vi "Do This.vi"(8 "error in (no error)":errorcluster, 10 "Status Events":refnum<class "Status Events.lvclass">, 11 "VI Analyzer in":refnum<class "VI Analyzer.lvclass">) -> (0 "error out":errorcluster, 3 "VI Analyzer out":refnum<class "VI Analyzer.lvclass">)   [LabVIEW 2014, in "VI Analyzer.lvclass"]
uses:
  VI Analyzer.lvclass
  Classes/Status Events/Status Events.lvclass
  Classes/Job/Job.lvclass/Job.ctl
  VI Analyzer.lvclass/VI Analyzer.ctl
  <vilib>/Utility/error.llb/DialogType.ctl
  <vilib>/addons/analyzer/NI_VIAnalyzerTKVIs.lvlib
  Classes/Job/Job.lvclass
  JUnit/VI Analyzer Parsing.lvlib
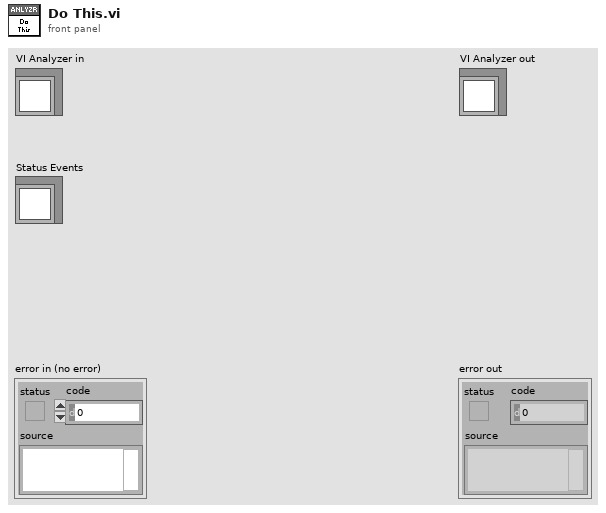
[diagram p1: front panel]
types:
  T1 = typedef "VIAnAPI Ref.ctl" = refnum<k1>
  T2 = typedef "VIAnCtl Results.ctl" = cluster{"Test Name":string, "Results Data":T3[], "Status":T4, "Exceed Max Fails?":bool}
  T3 = typedef "VIAnCtl ResultsData (index).ctl" = cluster{"Result Message":string, "Ref Index":i32}
  T4 = typedef "VIAnCtl ResultStatus.ctl" = enum16{"Pass", "Fail", "Skipped", "VI not loadable", "Test not loadable", "Test not runnable", "Test error out"}
  T5 = typedef "VIAnRes Parsed Results Data (by VI).ctl" = cluster{"VI Path":path, "Pass":cluster{"row":i32, "column":i32}[], "Fail":cluster{"row":i32, "column":i32}[], "Skipped":cluster{"row":i32, "column":i32}[], "VI not loadable":cluster{"row":i32, "column":i32}[], "Test not loadable":cluster{"row":i32, "column":i32}[], "Test not runnable":cluster{"row":i32, "column":i32}[], "Test error out":cluster{"row":i32, "column":i32}[]}
  T6 = typedef "VIAnRes Parsed Results Data (by Test).ctl" = cluster{"Test Name":string, "Pass":cluster{"VI Path":path, "index":cluster{"row":i32, "column":i32}}[], "Fail":cluster{"VI Path":path, "index":cluster{"row":i32, "column":i32}}[], "Skipped":cluster{"VI Path":path, "index":cluster{"row":i32, "column":i32}}[]}
  T7 = typedef "VIAnCtl Test Config Data.ctl" = cluster{"Test Name":string, "Config Ref":refnum<vi>, "Ref Valid?":bool, "Test Ranking":T8, "Max Failures":u32, "Test Path":path, "Control Values":T9[], "Selected?":bool}
  T8 = typedef "VIAnCtl TestRanking.ctl" = u16
  T9 = typedef "VIAnCtl Config Control Value.ctl" = cluster{"Control Name":string, "Control Value":variant}
  T10 = cluster{"Raw Results":T2[][], "Parsed Results Data (by VI)":T5[], "Parsed Results Data (by Test)":T6[], "Summary Statistics":cluster{"Passed Tests":i32, "Failed Tests":i32, "Skipped Tests":i32, "VIs not loadable":i32, "Tests not loadable":i32, "Tests not runnable":i32, "Test error out":i32, "Start Time":u32, "Total Time (s)":dbl}, "Test Config Data":T7[]}
  T11 = cluster{"Passed Tests":i32, "Failed Tests":i32, "Skipped Tests":i32, "VIs not loadable":i32, "Tests not loadable":i32, "Tests not runnable":i32, "Test error out":i32, "Start Time":u32, "Total Time (s)":dbl}
  T12 = typedef "DialogType.ctl" = u16
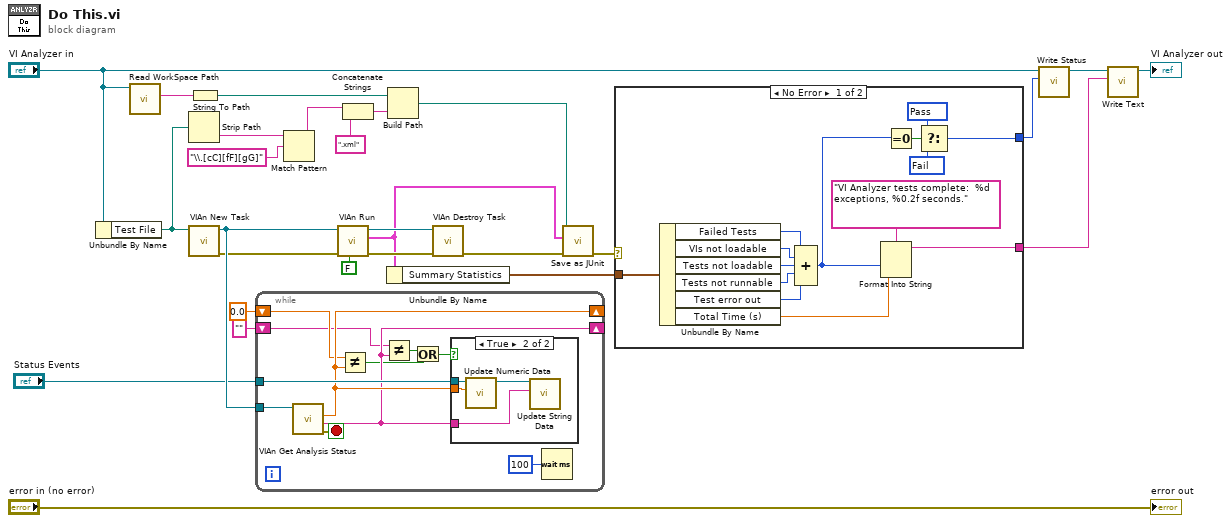
[diagram p0: block diagram]
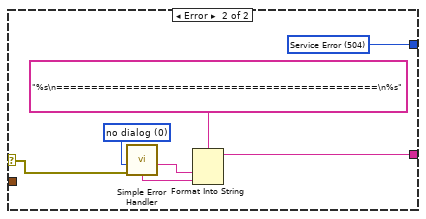
[diagram p2: hidden frame]
diagram:
  n1 = Unbundle By Name("VI Analyzer in") -> ("Test File"=w23:path)
  n2 = call "Read WorkSpace Path.vi"("Job in"="VI Analyzer in") -> ("WorkSpace Path"=w20:string)  [unwired: 8 in, 2 out]
  n3 = Strip Path(path=w23) -> (name=w21:string)  [unwired: 1 out]
  n4 = call <vilib>:"VIAn New Task.vi"("Path to Configuration File"=w23) -> ("error out"=w15:errorcluster, "VI Analyzer Task out"=w26:T1)  [unwired: 2 in, 7 out]
  n5 = String To Path(string=w20) -> (path=w19:path)
  n6 = while {
    tunnel: w26 -> [w36]
    tunnel: "Status Events" -> [w35]
    shift-right: [w34] -> _
    shift-left: 0.0 ("Percent Complete") -> [w33]
    shift-right: [w32] -> _
    shift-left: "" ("VI in Analysis") -> [w31]
    stop <- w37 stop-if-true
    n7 = call <vilib>:"VIAn Get Analysis Status.vi"("VI Analyzer Task in"=w36) -> ("error out"=w37:errorcluster, "VI in Analysis"=w32:string, "Percent Complete"=w34:dbl)  [unwired: 1 in, 7 out]
    n8 = Not Equal?(x=w33, y=w34) -> (x != y?=w29:bool)
    n9 = Not Equal?(x=w31, y=w32) -> (x != y?=w30:bool)
    n10 = Or(x=w30, y=w29) -> (x .or. y?=w28:bool)
    n11 = case shown="True" w28 {
      tunnel: w35 -> [_ w42]
      tunnel: w34 -> [_ w40]
      tunnel: w32 -> [_ w39]
      frame False {
      }
      frame True {
        n12 = call "Update Numeric Data.vi"("Numeric Data"=w40, "Status Updater in"=w42) -> ("Status Updater out"=w41:refnum<class "Status Events.lvclass">)  [unwired: 8 in, 1 out]
        n13 = call "Update String Data.vi"("String Data"=w39, "Status Updater in"=w41) -> ()  [unwired: 8 in, 2 out]
      }
    }
    n14 = Wait (ms)(milliseconds to wait=u32 100) -> ()  [unwired: 1 out]
  }
  n15 = Match Pattern(string=w21, regular expression="\\.[cC][fF][gG]") -> (before substring=w18:string)  [unwired: 1 in, 3 out]
  n16 = call <vilib>:"VIAn Run.vi"("Show Results Window?"=FALSE, "error in (no error)"=w15, "VI Analyzer Task in"=w26) -> ("error out"=w14:errorcluster, "Analysis Results"=w1:T10, "VI Analyzer Task out"=w27:T1)  [unwired: 6 out]
  n17 = Concatenate Strings(w18, ".xml" ("string")) -> (w8:string)
  n18 = Unbundle By Name(w1) -> ("Summary Statistics"=w16:T11)
  n19 = Build Path(base path=w19, name or relative path=w8) -> (appended path=w2:path)
  n20 = call <vilib>:"VIAn Destroy Task.vi"("error in (no error)"=w14, "VI Analyzer Task in"=w27) -> ("error out"=w3:errorcluster)  [unwired: 9 out]
  n21 = call "Save as JUnit.vi"("Error In (No Error)"=w3, "Analysis Results"=w1, "XML file path"=w2) -> ("Error Out"=w4:errorcluster)  [unwired: 8 in]
  n22 = case shown="No Error" w4 {
    selector: w4 -> [_ w58]
    tunnel: w16 -> [w56 _]
    tunnel: [w43 w63] -> w13
    tunnel: [w48 w57] -> w12
    frame No Error {
      w46 = u16 200 items=["Service Error"=504, "Abort"=503, "Fail"=500, "Pass"=200] ("Status")
      w47 = u16 500 items=["Service Error"=504, "Abort"=503, "Fail"=500, "Pass"=200] ("Status")
      n23 = Unbundle By Name(w56) -> ("Failed Tests"=w52:i32, "VIs not loadable"=w51:i32, "Tests not loadable"=w55:i32, "Tests not runnable"=w54:i32, "Test error out"=w53:i32, "Total Time (s)"=w49:dbl)
      n24 = Compound Arithmetic op=ADD(w52, w51, w55, w54, w53) -> (w45:i32)
      n25 = Format Into String(format string="VI Analyzer tests complete:  %d exceptions, %0.2f seconds.", w45, w49) -> (resulting string=w48:string)  [unwired: 2 in, 1 out]
      n26 = Equal To 0?(x=w45) -> (x = 0?=w44:bool)
      n27 = Select(t=w46, s=w44, f=w47) -> (s? t:f=w43:u16)
    }
    frame Error {
      w62 = T12 0 items=["no dialog", "OK message", "continue or stop message", "OK message + warnings", "continue/stop + warnings"] ("type of dialog (OK msg:1)")
      w63 = u16 504 items=["Service Error"=504, "Abort"=503, "Fail"=500, "Pass"=200] ("Status")
      n28 = call <vilib>:"Simple Error Handler.vi"("type of dialog (OK msg:1)"=w62, "error in (no error)"=w58) -> ("source out"=w60:string, "message"=w59:string)  [unwired: 3 in, 3 out]
      n29 = Format Into String(format string="%s\n==============================================\n%s", w60, w59) -> (resulting string=w57:string)  [unwired: 2 in, 1 out]
    }
  }
  n30 = call "Write Status.vi"("Status"=w13, "Job in"="VI Analyzer in") -> ("Job out"=w25:refnum<class "VI Analyzer.lvclass">)  [unwired: 8 in, 1 out]
  n31 = call "Write Text.vi"("Text"=w12, "Job in"=w25) -> ("Job out"=→"VI Analyzer out":refnum<class "VI Analyzer.lvclass">)  [unwired: 8 in, 1 out]
  "error out" <- "error in (no error)"
